vi "Append Report Text (str).vi"(0 "report in":refnum<class "ooWriter.lvclass">, 1 "MS Office parameters":T1, 2 "format string (%.3f)":string="%.3f", 7 "text":string, 9 "append on new line? (F)":bool, 11 "error in (no error)":errorcluster) -> (4 "report out":refnum<class "ooWriter.lvclass">, 8 "start out (Word)":i32, 10 "end out (Word)":i32, 15 "error out":errorcluster)   [LabVIEW 2009, in "ooWriter.lvclass"]
doc: "Appends text to the selected report."
uses:
  ooWriter.lvclass
  ooWriter.lvclass/ooWriter.ctl
  C:/Projets/LAVAG/OpenOfficeRGT/AODL/DLLs/AODL.dll
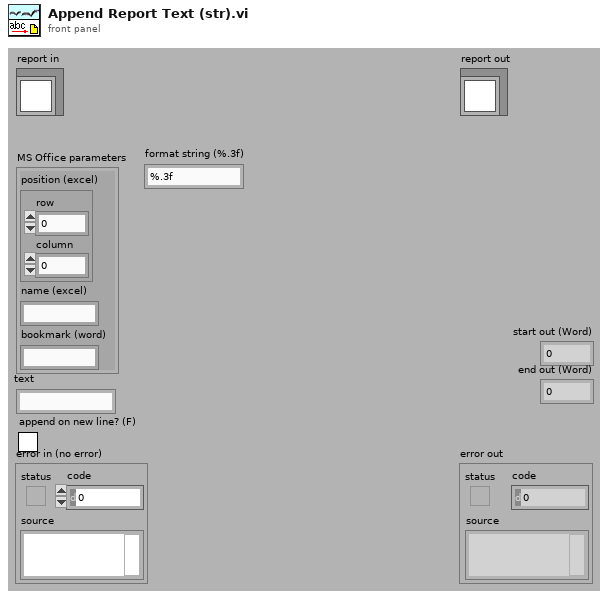
[diagram p1: front panel]
types:
  T1 = cluster{"position (excel)":cluster{"row":i32, "column":i32}, "name (excel)":string, "bookmark (word)":string}
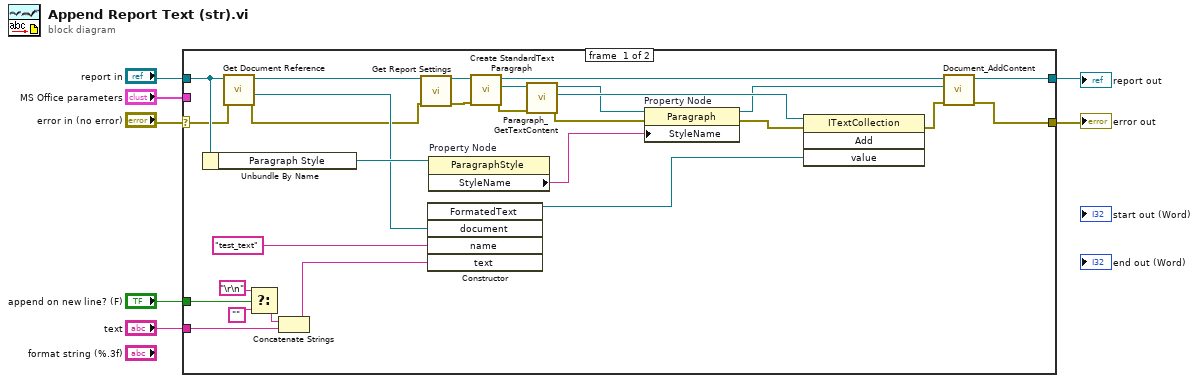
[diagram p0: block diagram]
diagram:
  n1 = case shown="No Error" "error in (no error)" {
    selector: "error in (no error)" -> [w9 w37]
    tunnel: [w13 w37] -> w5
    tunnel: [w31 w36] -> w6
    tunnel: "report in" -> [w11 w36]
    tunnel: "text" -> [w18 _]
    tunnel: "append on new line? (F)" -> [w35 _]
    tunnel: "MS Office parameters" -> [_ _]
    frame #0 {
      n2 = Unbundle By Name(w11) -> ("Paragraph Style"=w17:refnum<k24>)
      n3 = call-dynamic "Get Document Reference.vi"("error in (no error)"=w9, "ooDocument in"=w11) -> ("error out"=w8:errorcluster, "Document"=w12:refnum<k24>, "ooDocument out"=w10:refnum<class "ooWriter.lvclass">)  [unwired: 7 in]
      n4 = Select(t="\r\n", s=w35, f="") -> (s? t:f=w33:string)
      n5 = Concatenate Strings(w33, w18) -> (w25:string)
      n6 = call-dynamic "Get Report Settings.vi"("report in"=w10, "error in (no error)"=w8) -> ("report out"=w28:refnum<class "ooWriter.lvclass">, "error out"=w16:errorcluster)  [unwired: 9 in, 3 out]
      n7 = constructor class="FormatedText"("document"=w12, "name"="test_text", "text"=w25) -> (reference out=w30:refnum<k24>)  [unwired: 3 in, 5 out]
      n8 = property on="Property Node" class="ParagraphStyle"(reference=w17) -> ("StyleName"=w19:string)  [unwired: 1 in, 2 out]
      n9 = call-dynamic "Create StandardText Paragraph.vi"("error in (no error)"=w16, "ooWriter in"=w28) -> ("error out"=w15:errorcluster, "StandardTextParagraph"=w26:refnum<k24>, "ooWriter out"=w27:refnum<class "ooWriter.lvclass">)  [unwired: 7 in]
      n10 = call "Paragraph_GetTextContent.vi"("error in"=w15, "Paragraph"=w26) -> ("error out"=w14:errorcluster, "TextContent Collection"=w24:refnum<k24>, "Paragraph dup"=w22:refnum<k24>)  [unwired: 7 in]
      n11 = property on="Property Node" class="Paragraph"(reference=w22, error in=w14, "StyleName"=w19) -> (reference out=w21:refnum<k24>, error out=w20:errorcluster)
      n12 = invoke class="ITextCollection" method="Add"(reference=w24, error in=w20, "value"=w30) -> (error out=w29:errorcluster)  [unwired: 1 in, 3 out]
      n13 = call-dynamic "Document_AddContent.vi"("error in (no error)"=w29, "Content"=w21, "ooWriter in"=w27) -> ("error out"=w13:errorcluster, "ooWriter out"=w31:refnum<class "ooWriter.lvclass">)  [unwired: 7 in]
    }
    frame #1 {
    }
  }
  "error out" <- w5
  "report out" <- w6
